vi "Set Logging Timestamp in File Name.vi"(8 "error in":errorcluster, 10 "timestamp in file name":bool, 11 "logging in":T1=18446744073709551615 format="%.0x") -> (0 "error out":errorcluster, 3 "logging out":T1 format="%.0x")   [LabVIEW 2020, in "Ballard MIL-STD-1553 Scripting.lvlib"]
doc: "Specifies whether the log file name will be modified to contain a timestamp."
uses:
  <vilib>/NI VeriStand/Custom Device API/Custom Device Item Ref.ctl
  Constants.vi
  <vilib>/NI VeriStand/Custom Device API/Set Item Property (Boolean).vi
  Ballard MIL-STD-1553 Scripting.lvlib
  <vilib>/NI VeriStand/Custom Device API/Custom Device API.lvlib
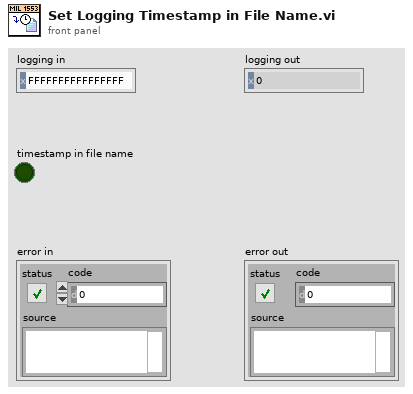
[diagram p1: front panel]
types:
  T1 = typedef "Custom Device API.lvlib/Custom Device Item Ref.ctl" = u64
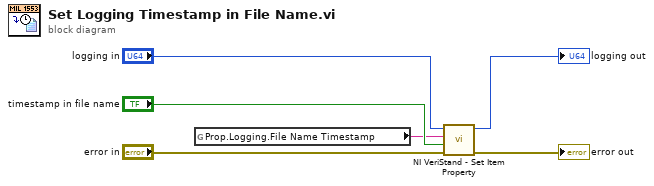
[diagram p0: block diagram]
diagram:
  n1 = global read "Constants.vi" "Prop.Logging.File Name Timestamp"() -> (w1:string)
  n2 = call-poly <vilib>:"NI VeriStand - Set Item Property.vi"("error in (no error)"="error in", "Value"="timestamp in file name", "Property Name"=w1, "Item Ref in"="logging in") -> ("error out"=→"error out":errorcluster, "Item Ref out"=→"logging out":T1)  [unwired: 5 in, 1 out]
